vi "Get component directory path.vi"(8 "error in (no error)":errorcluster, 10 "component specification":T1, 11 "ServiceManager in":refnum<class "ServiceManager.lvclass">) -> (0 "error out":errorcluster, 2 "path out":path, 3 "ServiceManager out":refnum<class "ServiceManager.lvclass">)   [LabVIEW 2012, in "ServiceManager.lvclass"]
uses:
  ServiceManager.lvclass
  <vilib>/Distrio/Murmex/Murmex/component_specification_cluster.ctl
  <vilib>/Distrio/Murmex/Murmex/Murmex.lvclass
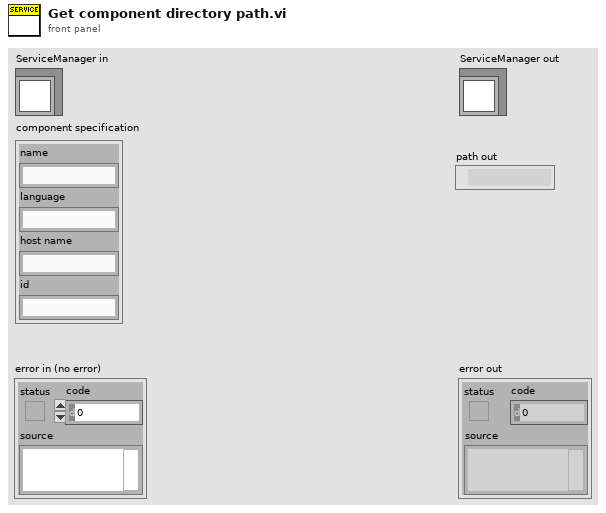
[diagram p1: front panel]
types:
  T1 = typedef "Murmex.lvlib/Murmex.lvclass/component_specification_cluster.ctl" = cluster{"name":string, "language":string, "host name":string, "id":string}
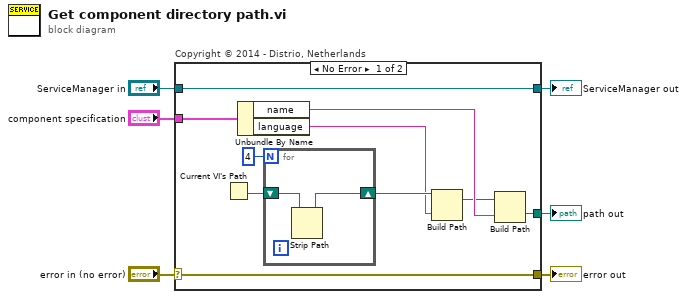
[diagram p0: block diagram]
diagram:
  n1 = case "Copyright © 2014 - Distrio, Netherlands" shown="No Error" "error in (no error)" {
    selector: "error in (no error)" -> [w15 w20]
    tunnel: [w15 w20] -> w5
    tunnel: [w16 w19] -> w3
    tunnel: "ServiceManager in" -> [w16 w19]
    tunnel: "component specification" -> [w14 _]
    tunnel: [w7 _] -> w1
    frame No Error {
      n2 = Current VI's Path() -> (path=w13:path)
      n3 = Unbundle By Name(w14) -> ("name"=w9:string, "language"=w10:string)
      n4 = for {
        N: 4 -> [_]
        shift-right: [w17] -> w11
        shift-left: w13 -> [w18]
        n5 = Strip Path(path=w18) -> (stripped path=w17:path)  [unwired: 1 out]
      }
      n6 = Build Path(base path=w11, name or relative path=w10) -> (appended path=w8:path)
      n7 = Build Path(base path=w8, name or relative path=w9) -> (appended path=w7:path)
    }
    frame Error {
    }
  }
  "error out" <- w5
  "ServiceManager out" <- w3
  "path out" <- w1
